vi "CalculateCRC.vi"(11 "data in":u8[](array[numeric])) -> (2 "CRC":u8, 3 "data out":u8[](array[numeric]))   [LabVIEW 2018]
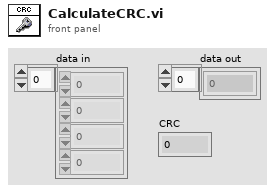
[diagram p1: front panel]
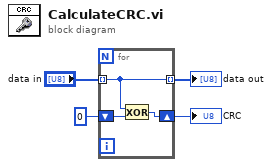
[diagram p0: block diagram]
diagram:
  n1 = for {
    tunnel: "data in" -> [w5] mode=indexing
    shift-right: [w6] -> w4
    shift-left: u8 0 -> [w7]
    tunnel: [w5] -> w3 mode=indexing
    n2 = Exclusive Or(1:w7, 2:w5) -> (0:w6:u8)
  }
  "CRC" <- w4
  "data out" <- w3
